vi "1.4.6-Lidar Encoder.vi"   [LabVIEW 2010]
uses:
  <vilib>/eio/EIONode/EIONode.xnode
  <vilib>/rvi/eio/nirviEIOImplementation/nirviEIOImplementation.xnode
  <vilib>/rvi/eio/common/nirviEmuClasses.ctl
  1.0-Hindbrain Global.vi
  <vilib>/rvi/eio/common/nirviEmuTemplateMethod_noerrors.vi
types:
  T1 = typedef "nirviEmuClasses.ctl" = enum16{"IO Read", "IO Write", "Method", "Property Read", "Property Write"}
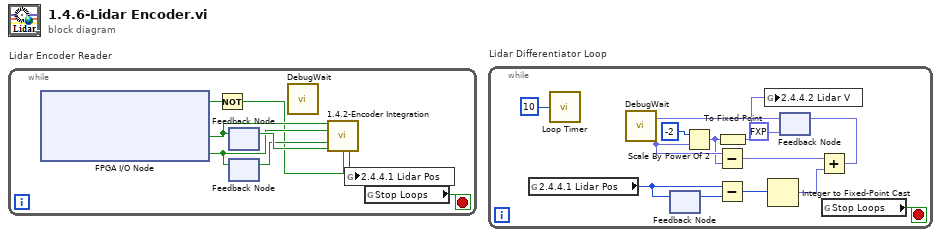
[diagram p0: block diagram]
diagram:
  n1 = while "Lidar Encoder Reader" {
    stop <- w8 stop-if-true
    n2 = xnode "FPGA I/O Node"() -> ("Lidar Pos Encoder Index"=w4:bool, "Lidar Pos Encoder B"=w5:bool, "Lidar Pos Encoder A"=w6:bool)  [unwired: 3 in, 3 out]
    n3 = Not(x=w4) -> (.not. x?=w1:bool)
    n4 = feedback #1() -> (w7:bool)  [unwired: 1 in]
    n5 = feedback-in #1(w5) -> ()
    n6 = feedback-in #2(w6) -> ()
    n7 = feedback #2() -> (w2:bool)  [unwired: 1 in]
    n8 = call "DebugWait.vi"() -> ()  [unwired: 12 in]
    n9 = call "1.4.2-Encoder Integration.vi"("Encoder B"=w5, "Encoder A"=w6, "Encoder A Old"=w2, "Encoder B Old"=w7, "Encoder Index"=w1) -> ("Current count"=w3:i32)  [unwired: 5 in, 5 out]
    n10 = global write "1.0-Hindbrain Global.vi" "2.4.4.1 Lidar Pos"(w3) -> ()
    n11 = global read "1.0-Hindbrain Global.vi" "Stop Loops"() -> (w8:bool)
  }
  n12 = while "Lidar Differentiator Loop" {
    stop <- w77 stop-if-true
    n13 = global read "1.0-Hindbrain Global.vi" "2.4.4.1 Lidar Pos"() -> (w76:i32)
    n14 = call "Loop Timer"("Count(mSec)"=u32 10 ("Count(Ticks)")) -> ()  [unwired: 1 out]
    n15 = call "DebugWait.vi"() -> ()  [unwired: 12 in]
    n16 = feedback #3() -> (w75:i32)  [unwired: 1 in]
    n17 = feedback-in #3(w76) -> ()
    n18 = Subtract(x=w76, y=w75) -> (x-y=w74:i32)
    n19 = Integer to Fixed-Point Cast(integer=w74) -> (fixed-point=w68:fxp<+/-,12,10>)  [unwired: 1 in]
    n20 = feedback #4(fxp<+/-,12,10> 0.0) -> (w70:fxp<+/-,12,10>)
    n21 = Scale By Power Of 2(n=i8 -2, x=w70) -> (x*2^n=w67:fxp<+/-,12,10>)
    n22 = Subtract(x=w70, y=w67) -> (x-y=w73:fxp<+/-,12,10>)
    n23 = To Fixed-Point(number=w67) -> (fixed-point=w66:fxp<+/-,10,8>)  [unwired: 1 in]
    n24 = global write "1.0-Hindbrain Global.vi" "2.4.4.2 Lidar V"(w66) -> ()
    n25 = Add(x=w73, y=w68) -> (x+y=w69:fxp<+/-,12,10>)
    n26 = feedback-in #4(w69) -> ()
    n27 = global read "1.0-Hindbrain Global.vi" "Stop Loops"() -> (w77:bool)
  }
